vi "Bad Setting Error.vi"(8 "error in (no error)":errorcluster, 9 "value":string, 10 "key":string, 11 "GE Reflective Memory Transceiver in":refnum<class "GE Reflective Memory Transceiver.lvclass">) -> (0 "error out":errorcluster, 3 "GE Reflective Memory Transceiver out":refnum<class "GE Reflective Memory Transceiver.lvclass">)   [LabVIEW 2017, in "GE Reflective Memory Transceiver.lvlib" / "GE Reflective Memory Transceiver.lvclass"]
uses:
  GE Reflective Memory Transceiver.lvclass
  <vilib>/NI/Memory Manager/VIs/New Error Cluster (512B).vi
  <vilib>/NI/Memory Manager/Static Errors.lvlib
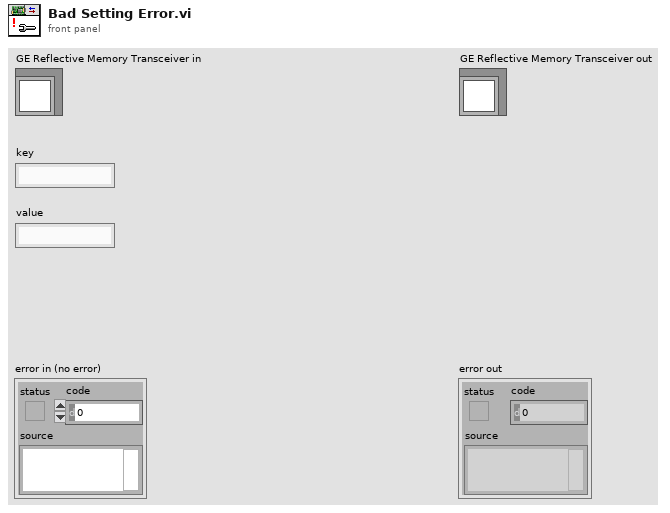
[diagram p1: front panel]
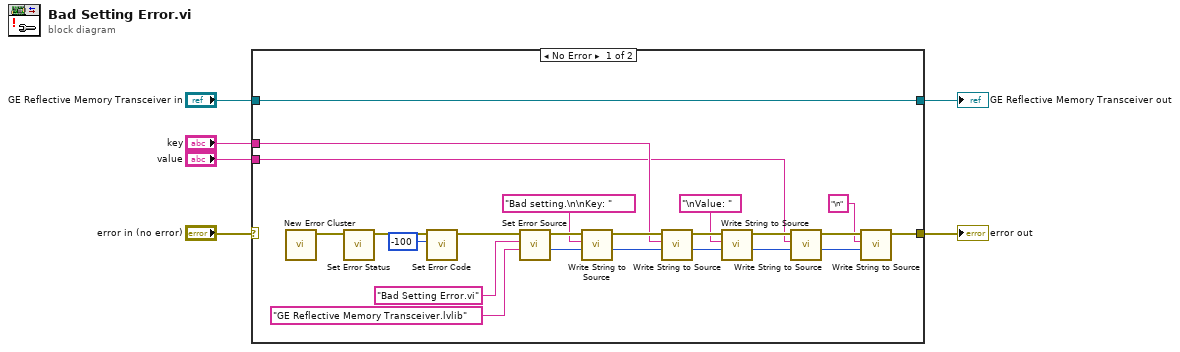
[diagram p0: block diagram]
diagram:
  n1 = case shown="No Error" "error in (no error)" {
    selector: "error in (no error)" -> [_ w31]
    tunnel: "key" -> [w17 _]
    tunnel: "value" -> [w11 _]
    tunnel: "GE Reflective Memory Transceiver in" -> [w27 w30]
    tunnel: [w27 w30] -> w3
    tunnel: [w9 w31] -> w1
    frame No Error {
      n2 = call-poly <vilib>:"New Error Cluster.vi"() -> ("error out"=w29:errorcluster)  [unwired: 10 in, 1 out]
      n3 = call <vilib>:"Set Error Status.vi"("error in"=w29) -> ("error out"=w28:errorcluster)  [unwired: 9 in, 1 out]
      n4 = call <vilib>:"Set Error Code.vi"("code"=-100, "error in"=w28) -> ("error out"=w25:errorcluster)  [unwired: 8 in, 1 out]
      n5 = call <vilib>:"Set Error Source.vi"("library name (\"\")"="GE Reflective Memory Transceiver.lvlib" ("library name (\"\")"), "vi name"="Bad Setting Error.vi", "error in"=w25) -> ("initial offset"=w21:i32, "error out"=w22:errorcluster)  [unwired: 7 in]
      n6 = call <vilib>:"Write String to Source.vi"("offset"=w21, "string"="Bad setting.\n\nKey: ", "error in"=w22) -> ("new offset"=w18:i32, "error out"=w19:errorcluster)  [unwired: 7 in]
      n7 = call <vilib>:"Write String to Source.vi"("offset"=w18, "string"=w17, "error in"=w19) -> ("new offset"=w14:i32, "error out"=w16:errorcluster)  [unwired: 7 in]
      n8 = call <vilib>:"Write String to Source.vi"("offset"=w14, "string"="\nValue: ", "error in"=w16) -> ("new offset"=w12:i32, "error out"=w13:errorcluster)  [unwired: 7 in]
      n9 = call <vilib>:"Write String to Source.vi"("offset"=w12, "string"=w11, "error in"=w13) -> ("new offset"=w8:i32, "error out"=w10:errorcluster)  [unwired: 7 in]
      n10 = call <vilib>:"Write String to Source.vi"("offset"=w8, "string"="\n", "error in"=w10) -> ("error out"=w9:errorcluster)  [unwired: 7 in, 1 out]
    }
    frame Error {
    }
  }
  "error out" <- w1
  "GE Reflective Memory Transceiver out" <- w3
